vi "Sort VI Ref Type.vi"(10 "Panel B":refnum<class "Panel.lvclass">, 11 "Panel A":refnum<class "Panel.lvclass">) -> (3 "A < B":bool)   [LabVIEW 2020, in "OOPanel.lvlib"]
uses:
  <vilib>/IlluminatedG/IG OOPanel/OOPanel/OOPanel.lvlib
  <vilib>/IlluminatedG/IG OOPanel/OOPanel/Panel/Panel.lvclass
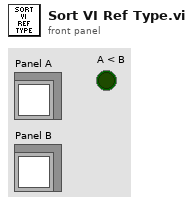
[diagram p1: front panel]
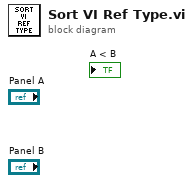
[diagram p0: block diagram]
diagram:
